vi "crossPoints.vi"() -> ()   [LabVIEW 2013]
uses:
  Data/TypeDefs/UTM Location.ctl
  Classes/Waypoint/Waypoint.lvclass
panel:
  in  "Irons Range":dbl=45.0
  in  "Absolute Wind Direction":dbl
  in  "Next Waypoint":refnum<class "Waypoint.lvclass">
  in  "Boat location":T1 {"North" format="%#_10f"; "East" format="%#_8f"}
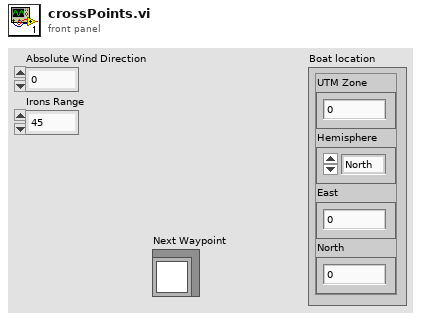
[diagram p1: front panel]
types:
  T1 = typedef "UTM Location.ctl" = cluster{"UTM Zone":dbl, "Hemisphere":enum16{"North", "South"}, "East":dbl, "North":dbl}
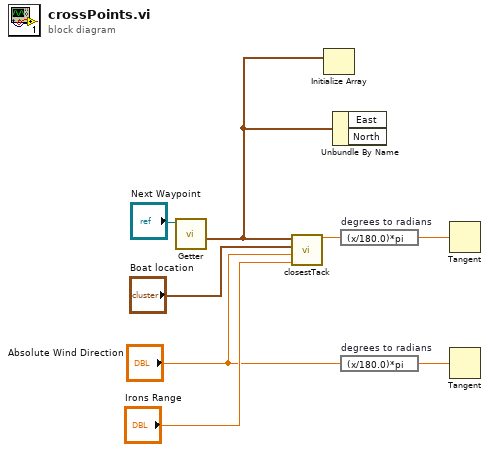
[diagram p0: block diagram]
diagram:
  n1 = call "Getter.vi"("Waypoint In"="Next Waypoint") -> ("Coords"=w1:T1)  [unwired: 6 in, 4 out]
  n2 = call "closestTack.vi"("Irons Range"="Irons Range", "Absolute Wind Direction"="Absolute Wind Direction", "Boat location"="Boat location", "PointA"=w1) -> ("closest tack"=w2:dbl)  [unwired: 7 in]
  n3 = Initialize Array(w1) -> ()  [unwired: 1 in, 1 out]
  n4 = Unbundle By Name(w1) -> ()  [unwired: 2 out]
  n5 = expression code="(x/180.0)*pi" "degrees to radians"(w2) -> (w3:dbl)
  n6 = expression code="(x/180.0)*pi" "degrees to radians"("Absolute Wind Direction") -> (w8:dbl)
  n7 = Tangent(1:w3) -> ()  [unwired: 1 out]
  n8 = Tangent(1:w8) -> ()  [unwired: 1 out]
